vi "PC_COUNT_ALL_Stations_for_month.vi"(0 "Refnum in":T1, 1 "data in":string[][](array[string]), 3 "Array 3":string[](array[string]), 5 "Select Month":string(combo), 7 "Select Year":string(combo), 11 "error in (no error)":errorcluster, 12 "STATION":i32[](array[numeric]), 14 "SHIFT":i32[](array[numeric])) -> (4 "Refnum out":T1, 6 "data out":string[][](array[string]), 8 "DATE":string[](array[string]), 10 "COUNT":string[](array[string]), 15 "error out":errorcluster)   [LabVIEW 2017]
uses:
  <vilib>/addons/database/Connection.llb/Conn ObjectReference.ctl
  <vilib>/addons/database/NI_Database_API.lvlib
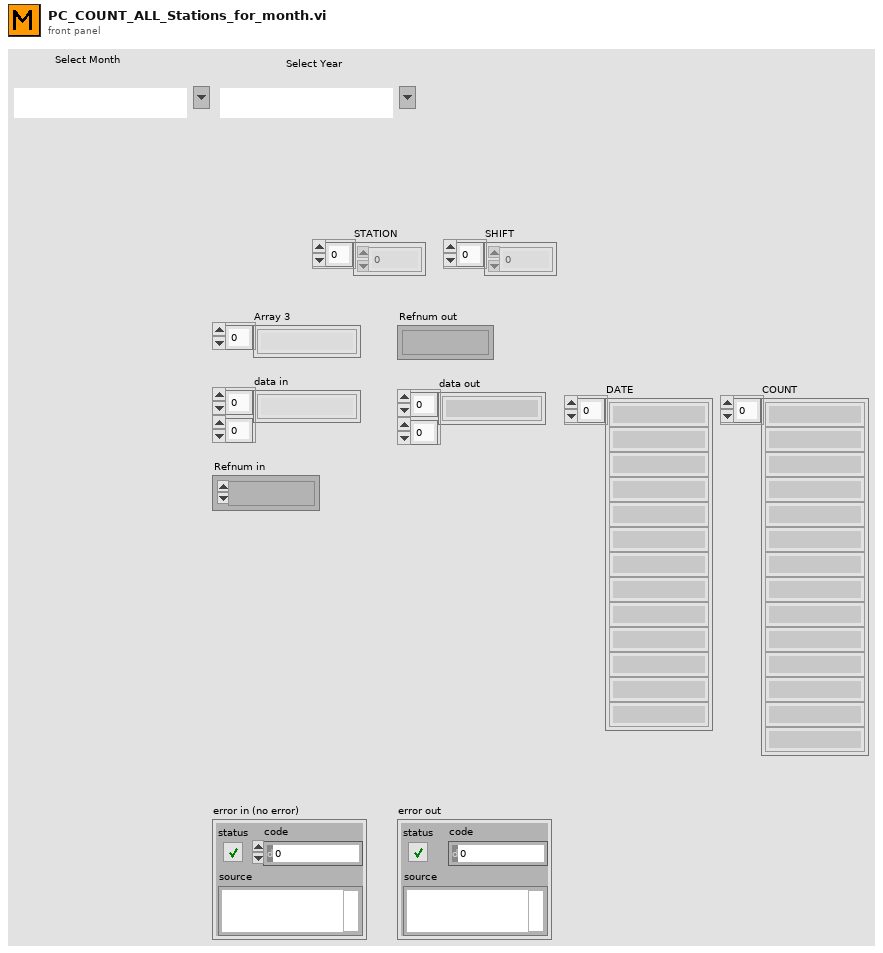
[diagram p1: front panel]
types:
  T1 = typedef "NI_Database_API.lvlib/Conn ObjectReference.ctl" = refnum<k1>
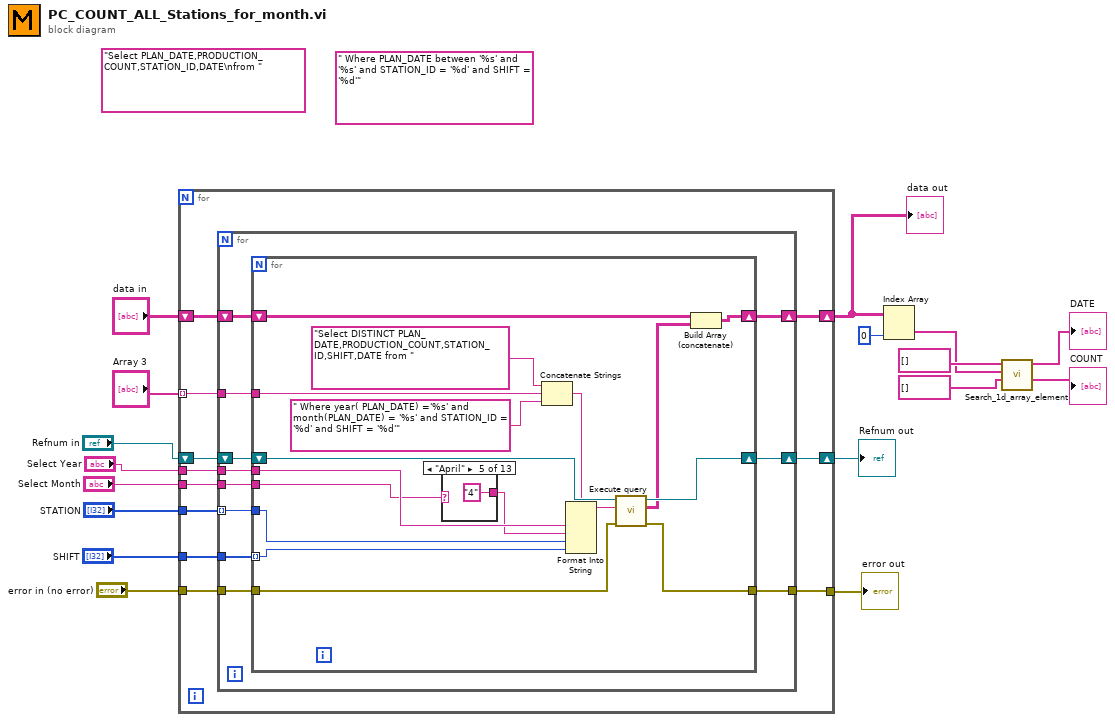
[diagram p0: block diagram]
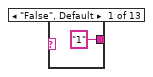
[diagram p2: hidden frame]
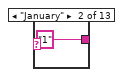
[diagram p3: hidden frame]
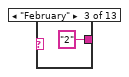
[diagram p4: hidden frame]
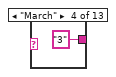
[diagram p5: hidden frame]
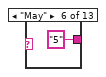
[diagram p6: hidden frame]
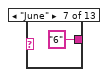
[diagram p7: hidden frame]
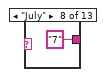
[diagram p8: hidden frame]
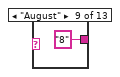
[diagram p9: hidden frame]
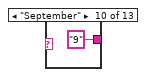
[diagram p10: hidden frame]
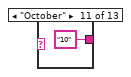
[diagram p11: hidden frame]
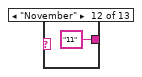
[diagram p12: hidden frame]
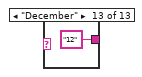
[diagram p13: hidden frame]
diagram:
  (unwired) " Where PLAN_DATE between '%s' and '%s' and STATION_ID = '%d' and SHIFT = '%d'"
  (unwired) "Select PLAN_DATE,PRODUCTION_COUNT,STATION_ID,DATE\nfrom "
  n1 = for {
    shift-right: [w27] -> w10
    shift-left: "Refnum in" -> [w28]
    tunnel: "Array 3" -> [w26] mode=indexing
    shift-right: [w22] -> w4
    shift-left: "data in" -> [w23]
    tunnel: "error in (no error)" -> [w25]
    tunnel: [w24] -> w14
    tunnel: "STATION" -> [w20]
    tunnel: "SHIFT" -> [w21]
    tunnel: "Select Year" -> [w19]
    tunnel: "Select Month" -> [w18]
    n2 = for {
      tunnel: w26 -> [w37]
      tunnel: w21 -> [w32]
      shift-right: [w38] -> w27
      shift-left: w28 -> [w39]
      shift-right: [w33] -> w22
      shift-left: w23 -> [w34]
      tunnel: w20 -> [w31] mode=indexing
      tunnel: w25 -> [w36]
      tunnel: [w35] -> w24
      tunnel: w19 -> [w30]
      tunnel: w18 -> [w29]
      n3 = for {
        tunnel: w37 -> [w54]
        shift-right: [w55] -> w38
        shift-left: w39 -> [w56]
        shift-right: [w50] -> w33
        shift-left: w34 -> [w51]
        tunnel: w32 -> [w44] mode=indexing
        tunnel: w31 -> [w45]
        tunnel: w36 -> [w53]
        tunnel: [w52] -> w35
        tunnel: w30 -> [w42]
        tunnel: w29 -> [w41]
        n4 = case shown="\"April\"" w41 {
          tunnel: ["1" "1" "2" "3" "4" "5" "6" "7" "8" "9" "10" "11" "12"] -> w40
          frame "False", Default {
          }
          frame "January" {
          }
          frame "February" {
          }
          frame "March" {
          }
          frame "April" {
          }
          frame "May" {
          }
          frame "June" {
          }
          frame "July" {
          }
          frame "August" {
          }
          frame "September" {
          }
          frame "October" {
          }
          frame "November" {
          }
          frame "December" {
          }
        }
        n5 = Concatenate Strings("Select DISTINCT PLAN_DATE,PRODUCTION_COUNT,STATION_ID,SHIFT,DATE from ", w54, " Where year( PLAN_DATE) ='%s' and month(PLAN_DATE) = '%s' and STATION_ID = '%d' and SHIFT = '%d'") -> (w48:string)
        n6 = Format Into String(format string=w48, w42, w40, w45, w44) -> (resulting string=w49:string)  [unwired: 2 in, 1 out]
        n7 = call "Execute query.vi"("error in (no error)"=w53, "String"=w49, "connection reference"=w56) -> ("error out"=w52:errorcluster, "Table"=w46:string[][], "connection reference 2"=w55:T1)  [unwired: 5 in, 1 out]
        n8 = Build Array (concatenate)(w51, w46) -> (w50:string[][])
      }
    }
  }
  "data out" <- w4
  "error out" <- w14
  "Refnum out" <- w10
  n9 = Index Array(array=w4, index (col)=0 ("disabled index (col)")) -> (element=w7:string[])  [unwired: 1 in]
  n10 = call "Search_1d_array_element.vi"("Count in"=string[] [] ("Count"), "BD Date"=w7, "Elements Found in"=string[] [] ("Elements Found")) -> ("Count out"=→"COUNT":string[], "Elements Found out"=→"DATE":string[])  [unwired: 4 in, 1 out]
